vi "[SubVI]DCvsVoltage.vi"(1 "Right Voltage Read":dbl, 2 "Right Duty Cycle":dbl, 3 "Right Motor Direction":bool, 8 "Left Voltage Read":dbl, 9 "Left Duty Cycle":dbl, 10 "Left Motor Direction":bool) -> (0 "Right cluster":T1, 7 "Left cluster":T1)   [LabVIEW 2018]
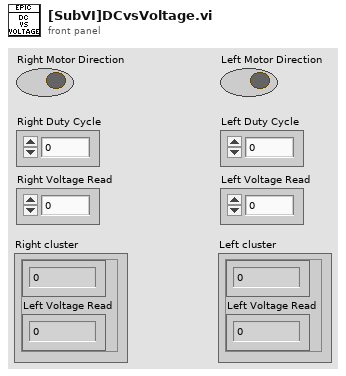
[diagram p1: front panel]
types:
  T1 = cluster{"Numeric Control":dbl, "Left Voltage Read":dbl}
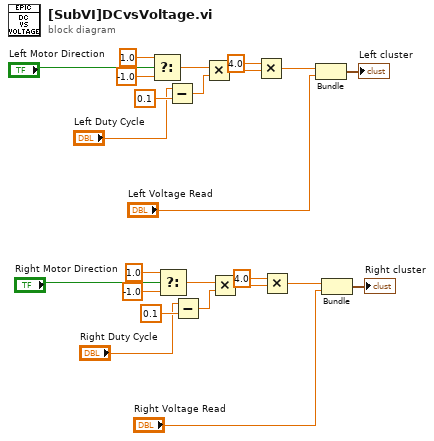
[diagram p0: block diagram]
diagram:
  n1 = Select(t=1.0, s="Left Motor Direction", f=-1.0) -> (s? t:f=w20:dbl)
  n2 = Select(t=1.0, s="Right Motor Direction", f=-1.0) -> (s? t:f=w8:dbl)
  n3 = Subtract(x="Left Duty Cycle", y=0.1) -> (x-y=w21:dbl)
  n4 = Subtract(x="Right Duty Cycle", y=0.1) -> (x-y=w9:dbl)
  n5 = Multiply(x=w20, y=w21) -> (x*y=w23:dbl)
  n6 = Multiply(x=w8, y=w9) -> (x*y=w11:dbl)
  n7 = Multiply(x=4.0, y=w23) -> (x*y=w17:dbl)
  n8 = Multiply(x=4.0, y=w11) -> (x*y=w5:dbl)
  n9 = Bundle(w17, "Left Voltage Read"="Left Voltage Read") -> (→"Left cluster":cluster{dbl, "Left Voltage Read":dbl})  [unwired: 1 in]
  n10 = Bundle(w5, "Right Voltage Read"="Right Voltage Read") -> (→"Right cluster":cluster{dbl, "Right Voltage Read":dbl})  [unwired: 1 in]
